vi "addXMLNode.vi"(8 "error in (no error)":errorcluster, 10 "LabVIEW Object":refnum<class>, 11 "xmlNode in":refnum<class "xmlNode.lvclass">) -> (0 "error out":errorcluster, 3 "xmlNode out":refnum<class "xmlNode.lvclass">)   [LabVIEW 2011, in "Tools.lvlib" / "xml.lvlib" / "xmlNode.lvclass"]
uses:
  xmlNode.lvclass
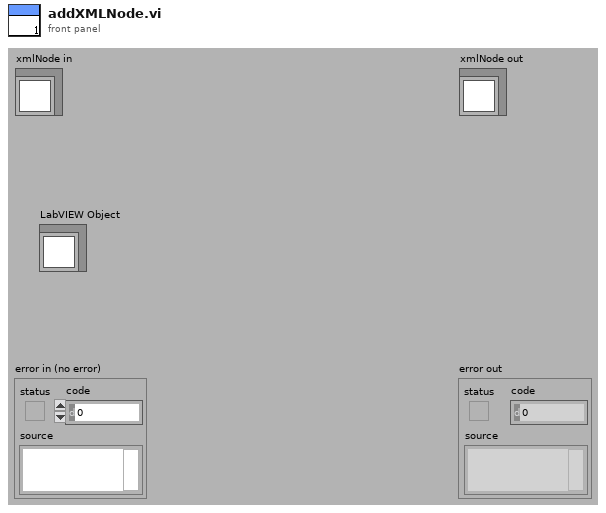
[diagram p1: front panel]
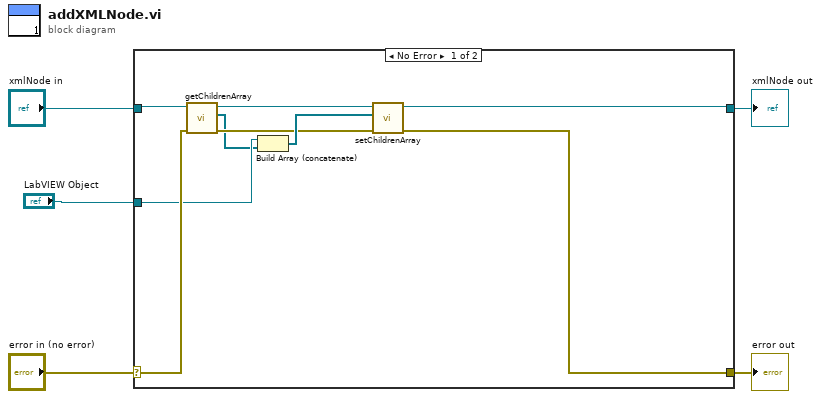
[diagram p0: block diagram]
diagram:
  n1 = case shown="No Error" "error in (no error)" {
    selector: "error in (no error)" -> [w13 w16]
    tunnel: [w9 w16] -> w4
    tunnel: [w8 w15] -> w2
    tunnel: "xmlNode in" -> [w14 w15]
    tunnel: "LabVIEW Object" -> [w7 _]
    frame No Error {
      n2 = call-dynamic "getChildrenArray.vi"("error in (no error)"=w13, "xmlNode.lvclass in"=w14) -> ("error out"=w10:errorcluster, "Children"=w6:refnum<class "xmlNode.lvclass">[], "xmlNode.lvclass out"=w11:refnum<class "xmlNode.lvclass">)  [unwired: 7 in]
      n3 = Build Array (concatenate)(w7, w6) -> (w12:refnum<class>[])
      n4 = call-dynamic "setChildrenArray.vi"("error in (no error)"=w10, "Children"=w12, "xmlNode.lvclass in"=w11) -> ("error out"=w9:errorcluster, "xmlNode.lvclass out"=w8:refnum<class "xmlNode.lvclass">)  [unwired: 7 in]
    }
    frame Error {
    }
  }
  "error out" <- w4
  "xmlNode out" <- w2
